vi "Number of Address Map Elements.vi"(2 "Basecard Config Registers":refnum<class "7902R Basecard Config Registers.lvclass">) -> (6 "number of elements":u8)   [LabVIEW 2019, in "7902R Basecard Config Registers.lvclass"]
uses:
  7902R Basecard Config Registers.lvclass
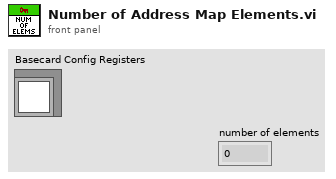
[diagram p1: front panel]
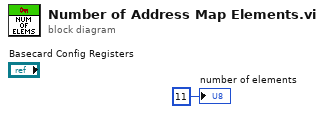
[diagram p0: block diagram]
diagram:
  "number of elements" <- u8 11 ("number of elements")
